vi "SetCursorPos(x,y)diagram.vi"(0 "vi reference":refnum<vi>, 5 "(X,Y)":T1, 7 "Xadjustment":i32=6, 9 "Yadjustment":i32=78, 11 "Error in":errorcluster) -> (4 "Sucess?":i32, 15 "Error out":errorcluster)   [LabVIEW 2013]
uses:
  <vilib>/Utility/miscctls.llb/LVPointTypeDef.ctl
  <vilib>/Utility/miscctls.llb/LVPositionTypeDef.ctl
  user32.dll
  Linux VIs/guiLib.so
panel:
  # "Any chages to the\n- name & path of this VI\n- Label name of 'Xadjustment' and 'Yadjustment' constants \nshould be reflected in the VI \"DetermineXYAdjustment.vi\""
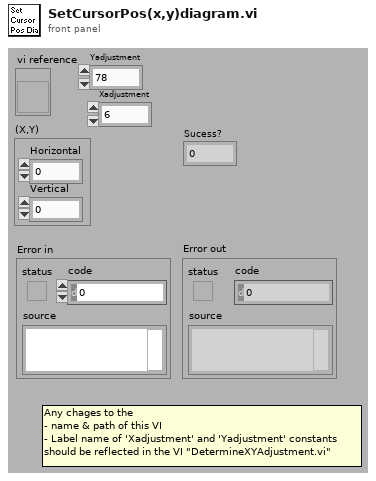
[diagram p1: front panel]
types:
  T1 = typedef "LVPointTypeDef.ctl" = cluster{"Horizontal":i16, "Vertical":i16}
  T2 = typedef "LVPositionTypeDef.ctl" = cluster{"Left":i32, "Top":i32}
  T3 = typedef "LVRectTypeDef.ctl" = cluster{"Left":i16, "Top":i16, "Right":i16, "Bottom":i16}
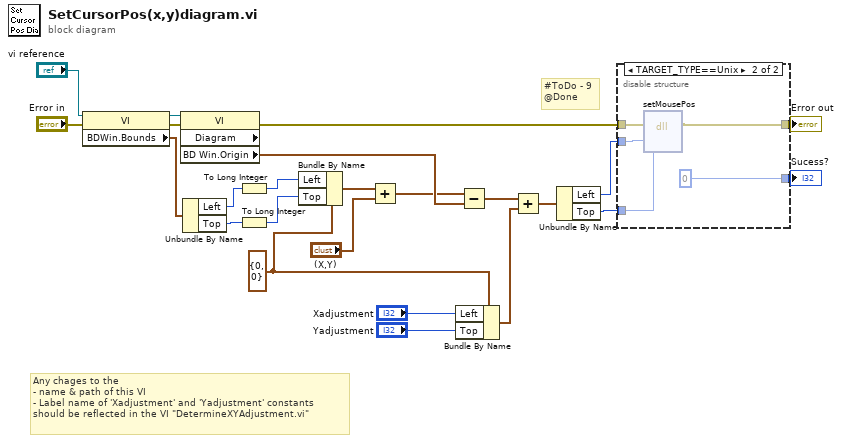
[diagram p0: block diagram]
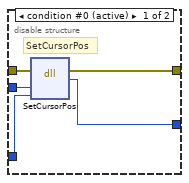
[diagram p2: hidden frame]
diagram:
  w16 = T2 {"Left"=0, "Top"=0} ("Position")
  # "#ToDo - 9\n@Done"
  # "Any chages to the\n- name & path of this VI\n- Label name of 'Xadjustment' and 'Yadjustment' constants \nshould be reflected in the VI \"DetermineXYAdjustment.vi\""
  n1 = property class="VI"(reference="vi reference", error in="Error in") -> (reference out=w2:refnum<vi>, error out=w1:errorcluster, "BDWin.Bounds"=w3:T3)
  n2 = property class="VI" props=["Diagram", "BD Win.Origin"](reference=w2, error in=w1) -> (error out=w12:errorcluster, "BD Win.Origin"=w15:T1)  [unwired: 2 out]
  n3 = Unbundle By Name(w3) -> ("Left"=w7:i16, "Top"=w10:i16)
  n4 = To Long Integer(number=w7) -> (32bit integer=w8:i32)
  n5 = To Long Integer(number=w10) -> (32bit integer=w9:i32)
  n6 = Bundle By Name(cluster=w16, "Left"=w8, "Top"=w9) -> (w4:T2)
  n7 = Add(x=w4, y="(X,Y)") -> (x+y=w14:T2)
  n8 = Bundle By Name(cluster=w16, "Left"="Xadjustment", "Top"="Yadjustment") -> (w19:T2)
  n9 = Subtract(x=w14, y=w15) -> (x-y=w20:T2)
  n10 = Add(x=w20, y=w19) -> (x+y=w21:T2)
  n11 = Unbundle By Name(w21) -> ("Left"=w5:i32, "Top"=w6:i32)
  n12 = disable-structure shown="TARGET_TYPE==Unix" {
    disable-tunnel: [w29 w34] -> w24
    disable-tunnel: w12 -> [w28 w33]
    disable-tunnel: [w27 0 ("Sucess?")] -> w11
    disable-tunnel: w6 -> [w26 w31]
    disable-tunnel: w5 -> [w25 w32]
    frame condition #0 (active) {
      # "SetCursorPos"
      n13 = dll-call lib="user32.*" fn="SetCursorPos"(error in=w28, "X"=w25, "Y"=w26) -> (error out=w29:errorcluster, "return type"=w27:i32)  [unwired: 4 in, 1 out]
    }
    frame condition #1 {
      n14 = dll-call lib="home/lvadmin/inmathed_linux_GUI/inmathed_linux_GUI/LabVIEWTestSystems/LV GUI ToolKit/LV GUI 2013/LabVIEW GUI Automation Toolkit/Utility/Linux VIs/guiLib.so" fn="setMousePos"(error in=w33, "X_axis"=w32, "Y_axis"=w31) -> (error out=w34:errorcluster)  [unwired: 5 in, 1 out]
    }
  }
  "Error out" <- w24
  "Sucess?" <- w11
